vi "Prod - Uninitialize.vi"(8 "Error In":errorcluster, 11 "Prod-Data In":T2={"Queue_Producer"=refnum, "Queue_Consumer"=refnum, "To_GUI-Error_message"=refnum, "Rx-Data"=[], "Tx-Data"=[], "Console log"="", "Communication Settings"={"Tx Protocol"=enum."Not Active", "Rx Protocol"=enum."Serial", "Serial"={"Tx Port"="", "Rx Port"="", "Baud rate"=8, "Parity"=enum."Space", "Data bits"=0, "Stop bits"=0, "Flow control"=enum."None", "Tx Resource"="", "Rx Resource"=""}, "MIDI Device"={"Input uDevice ID"=0, "Output uDevice ID"=0, "hmidiout Handle"=0, "hmidiin Handle"=0}, "Bluetooth"={"Dummy"=""}, "USB"={"Dummy"=""}}, "MIDI-Messages"=[], "Queue_Session"=refnum, "To_GUI-Pre-Session"=refnum, "To_GUI-Producer"=refnum, "Tx Info"={"Datatype"=[], "Bytesize"=[], "Strings"=[], "ByteSum"=0}, "Payload"=variant, "Timout-Time[ms]"=0, "To_GUI-Session"=refnum, "CPU(ms)"=0}) -> (0 "Error Out":errorcluster, 3 "Prod-Data Out":T2={"Queue_Producer"=refnum, "Queue_Consumer"=refnum, "To_GUI-Error_message"=refnum, "Rx-Data"=[], "Tx-Data"=[], "Console log"="", "Communication Settings"={"Tx Protocol"=enum."Not Active", "Rx Protocol"=enum."Serial", "Serial"={"Tx Port"="", "Rx Port"="", "Baud rate"=8, "Parity"=enum."Space", "Data bits"=0, "Stop bits"=0, "Flow control"=enum."None", "Tx Resource"="", "Rx Resource"=""}, "MIDI Device"={"Input uDevice ID"=0, "Output uDevice ID"=0, "hmidiout Handle"=0, "hmidiin Handle"=0}, "Bluetooth"={"Dummy"=""}, "USB"={"Dummy"=""}}, "MIDI-Messages"=[], "Queue_Session"=refnum, "To_GUI-Pre-Session"=refnum, "To_GUI-Producer"=refnum, "Tx Info"={"Datatype"=[], "Bytesize"=[], "Strings"=[], "ByteSum"=0}, "Payload"=variant, "Timout-Time[ms]"=0, "To_GUI-Session"=refnum, "CPU(ms)"=0})   [LabVIEW 2019]
doc: "Initiates the producer based on IO settings."
uses:
  Controls/Producer-Data.ctl
  Common/Controls/Application_Message.ctl
  Common/Controls/Application_State.ctl
  Common/Controls/Communication_Settings.ctl
  Common/Controls/Communication_Protocols.ctl
  MIDI/Controls/MIDI-Message_Array.ctl
  MIDI/Controls/MIDI-Message_Cluster.ctl
  MIDI/Controls/Meta_Commands.ctl
  Controls/Prod - Tx_Info.ctl
  <vilib>/Utility/error.llb/DialogType.ctl
  winmm.dll
panel:
  in  "Control Tab":T1(tab)
  out "Console":string
  out "Error Message":string
  out "VI-filename":string
  out "VI Path":path
  out "Code Size":u32
  out "Revision Number":u32
  in  "Tool Bar:Visible":bool
  in  "Execution:Show Front Panel On Call":bool
  out "VI-Name":string
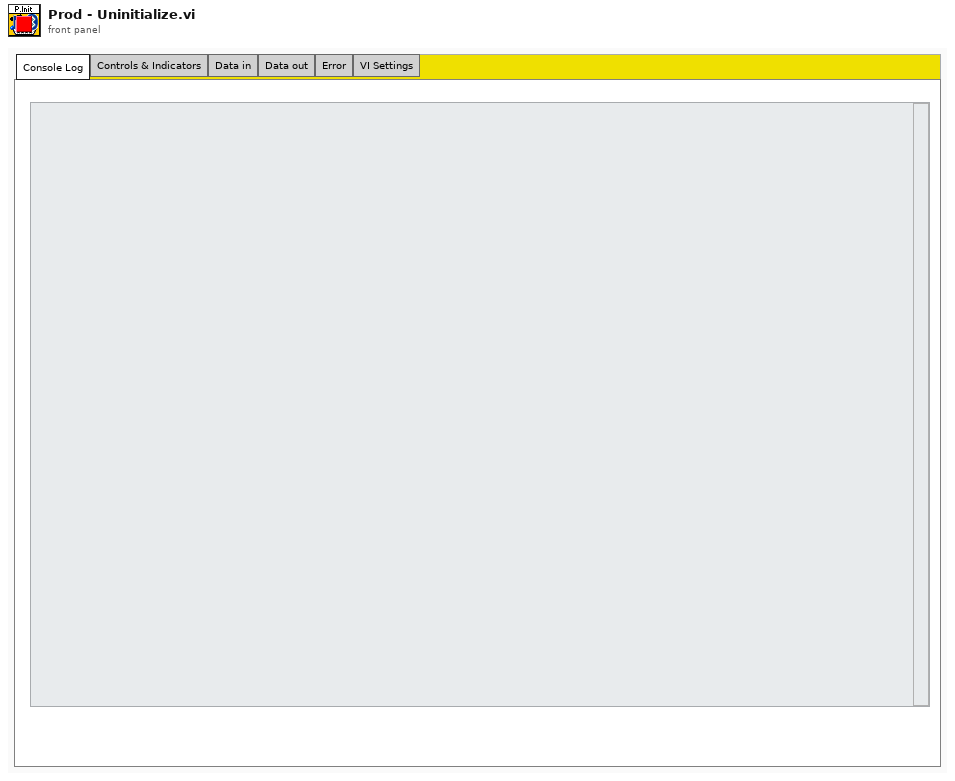
[diagram p1: front panel]
types:
  T1 = enum32{"Console Log", "Controls & Indicators", "Data in", "Data out", "Error", "VI Settings"}
  T2 = typedef "Producer-Data.ctl" = cluster{"Queue_Producer":refnum<queue>, "Queue_Consumer":refnum<queue>, "To_GUI-Error_message":refnum<user-event>, "Rx-Data":i8[], "Tx-Data":i8[], "Console log":string, "Communication Settings":T3, "MIDI-Messages":T5, "Queue_Session":refnum<queue>, "To_GUI-Pre-Session":refnum<user-event>, "To_GUI-Producer":refnum<user-event>, "Tx Info":T8, "Payload":variant, "Timout-Time[ms]":i32, "To_GUI-Session":refnum<user-event>, "CPU(ms)":u32}
  T3 = typedef "Communication_Settings.ctl" = cluster{"Tx Protocol":T4, "Rx Protocol":T4, "Serial":cluster{"Tx Port":refnum<visa-resource-name>, "Rx Port":refnum<visa-resource-name>, "Baud rate":i32, "Parity":enum16{"None", "Odd", "Even", "Mark", "Space"}, "Data bits":i32, "Stop bits":i32, "Flow control":enum16{"None", "XON/XOFF", "RTS/CTS", "XON/XOFF & RTS/CTS", "DTR/DSR", "XON/XOFF & DTR/DSR"}, "Tx Resource":refnum<visa-resource-name>, "Rx Resource":refnum<visa-resource-name>}, "MIDI Device":cluster{"Input uDevice ID":u32, "Output uDevice ID":u32, "hmidiout Handle":i32, "hmidiin Handle":i32}, "Bluetooth":cluster{"Dummy":string}, "USB":cluster{"Dummy":string}}
  T4 = typedef "Communication_Protocols.ctl" = enum16{"Serial", "Bluetooth", "USB-MIDI", "MIDI (Audio Device)", "Not Active"}
  T5 = typedef "MIDI-Message_Array.ctl" = T6[]
  T6 = typedef "MIDI-Message_Cluster.ctl" = cluster{"Message Name":string, "Meta value":i32, "Datastring":string, "Datatype":T7}
  T7 = typedef "Meta_Commands.ctl" = enum16{"No Data", "Pause", "Loop", "Wait for Rx", "Delay", "Break", "MIDI"}
  T8 = typedef "Prod - Tx_Info.ctl" = cluster{"Datatype":T7[], "Bytesize":i32[], "Strings":string[], "ByteSum":i32}
  T9 = typedef "DialogType.ctl" = u16
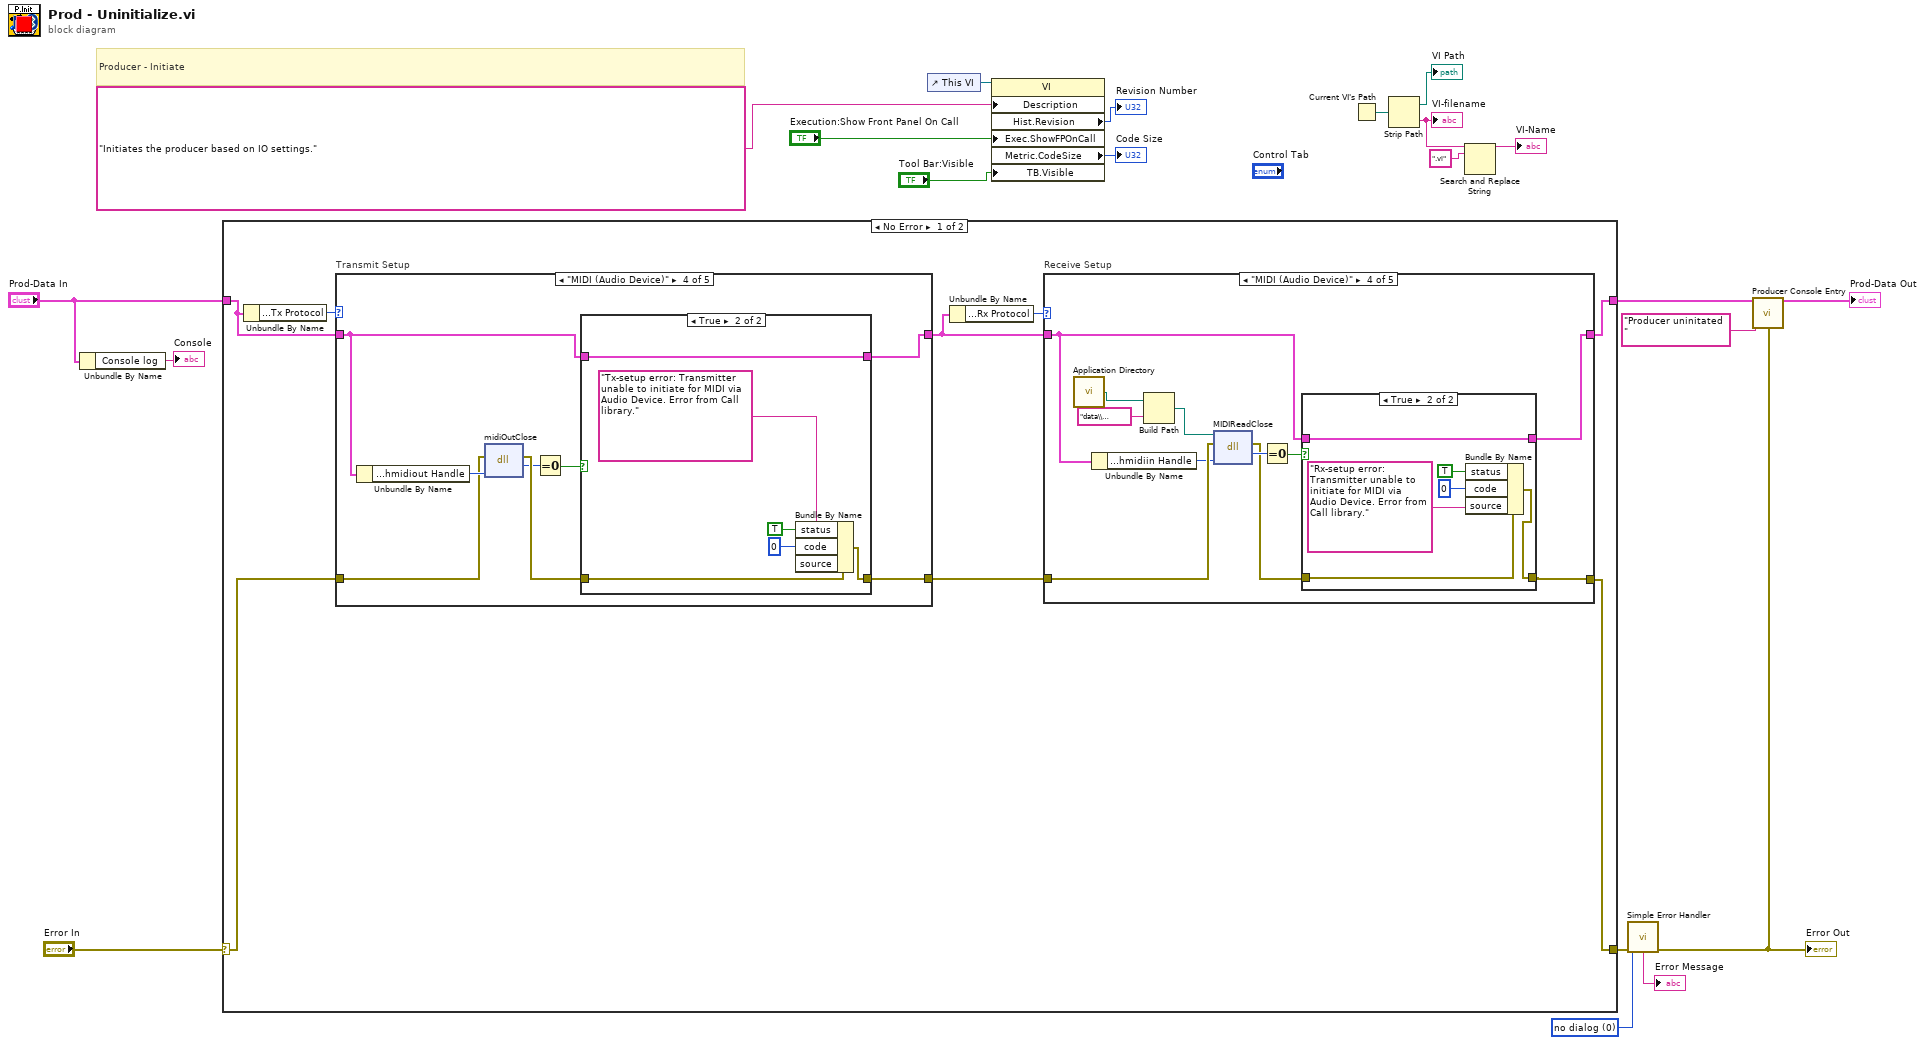
[diagram p0: block diagram]
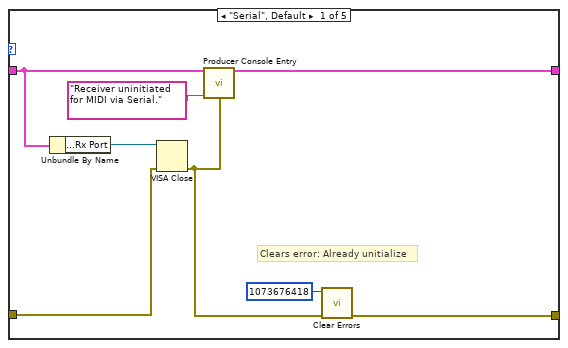
[diagram p2: hidden frame]
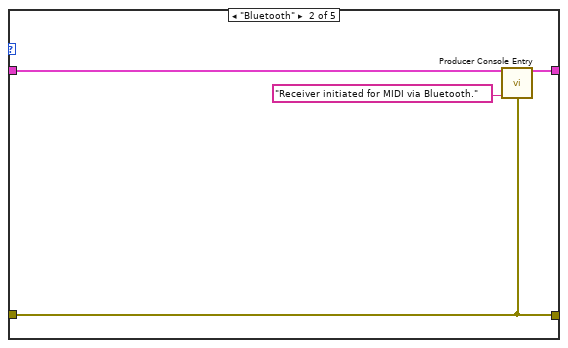
[diagram p3: hidden frame]
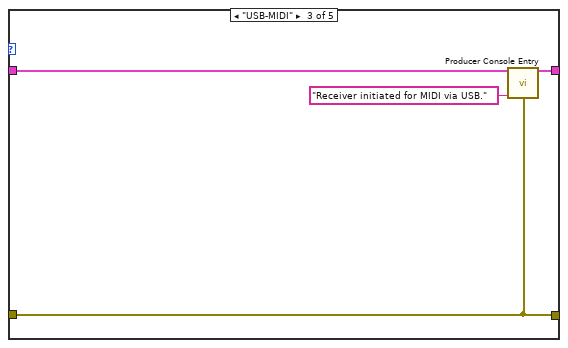
[diagram p4: hidden frame]
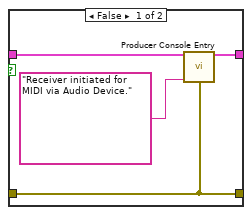
[diagram p5: hidden frame]
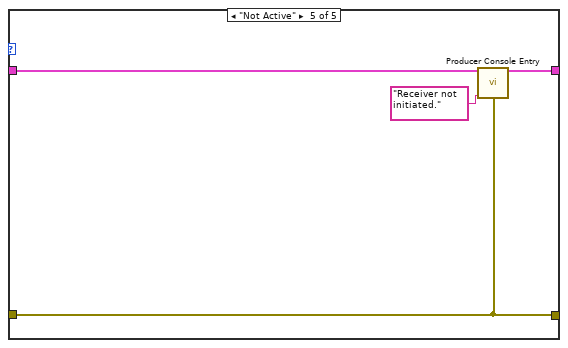
[diagram p6: hidden frame]
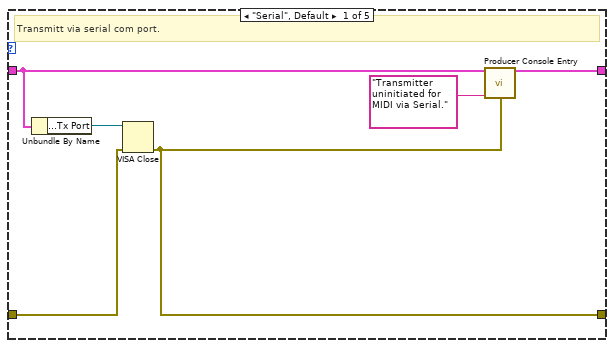
[diagram p7: hidden frame]
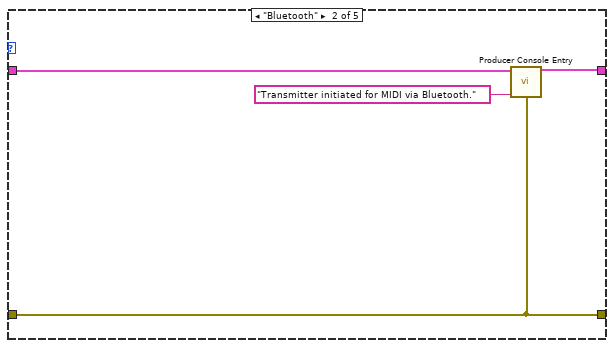
[diagram p8: hidden frame]
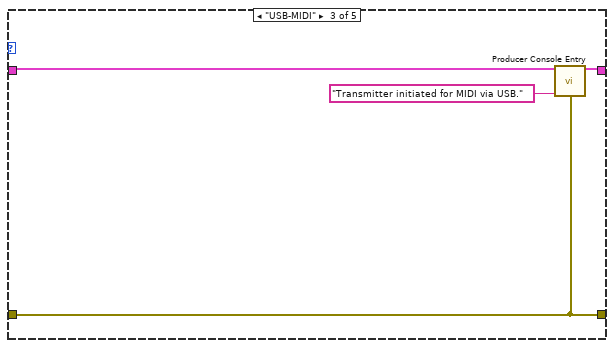
[diagram p9: hidden frame]
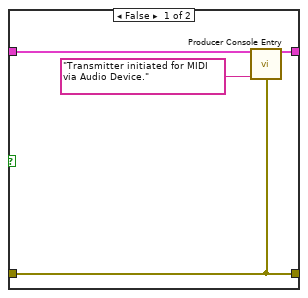
[diagram p10: hidden frame]
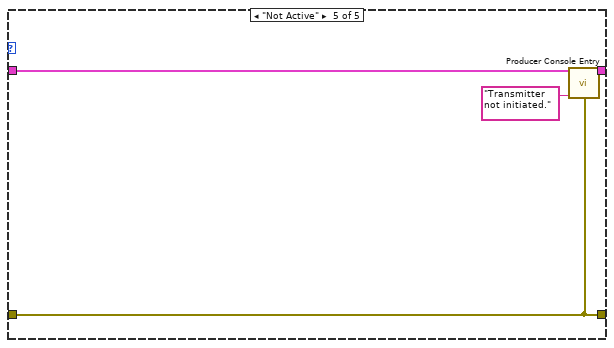
[diagram p11: hidden frame]
diagram:
  w4 = T9 0 items=["no dialog", "OK message", "continue or stop message", "OK message + warnings", "continue/stop + warnings"] ("type of dialog (OK msg:1)")
  # "Producer - Initiate"
  n1 = Unbundle By Name("Prod-Data In") -> ("Console log"=→"Console":string)
  n2 = case shown="No Error" "Error In" {
    selector: "Error In" -> [w24 w108]
    tunnel: [w22 w108] -> w6
    tunnel: "Prod-Data In" -> [w28 w107]
    tunnel: [w25 w107] -> w7
    frame No Error {
      n3 = Unbundle By Name(w28) -> ("Communication Settings.Tx Protocol"=w29:T4)
      n4 = case "Transmit Setup" shown="\"MIDI (Audio Device)\"" w29 {
        tunnel: w28 -> [w76 w78 w82 w85 w105]
        tunnel: [w75 w80 w83 w86 w106] -> w26
        tunnel: w24 -> [w72 w79 w81 w91 w103]
        tunnel: [w71 w79 w81 w89 w103] -> w23
        frame "Serial", Default {
          # "Transmitt via serial com port."
          n5 = Unbundle By Name(w76) -> ("Communication Settings.Serial.Tx Port"=w73:refnum<visa-resource-name>)
          n6 = VISA Close(VISA resource name=w73, error in (no error)=w72) -> (error out=w71:errorcluster)
          n7 = call "Producer Console Entry.vi"("Prod-Data In"=w76, "Console Entry"="Transmitter uninitiated for MIDI via Serial.", "Error In"=w71) -> ("Prod-Data Out"=w75:T2)  [unwired: 12 in]
        }
        frame "Bluetooth" {
          n8 = call "Producer Console Entry.vi"("Prod-Data In"=w78, "Console Entry"="Transmitter initiated for MIDI via Bluetooth.", "Error In"=w79) -> ("Prod-Data Out"=w80:T2)  [unwired: 12 in]
        }
        frame "USB-MIDI" {
          n9 = call "Producer Console Entry.vi"("Prod-Data In"=w82, "Console Entry"="Transmitter initiated for MIDI via USB.", "Error In"=w81) -> ("Prod-Data Out"=w83:T2)  [unwired: 12 in]
        }
        frame "MIDI (Audio Device)" {
          n10 = Unbundle By Name(w85) -> ("Communication Settings.MIDI Device.hmidiout Handle"=w92:i32)
          n11 = dll-call lib="winmm.dll" fn="midiOutClose"(error in=w91, "hmidiout"=w92) -> (error out=w90:errorcluster, w88:i32)  [unwired: 3 in, 1 out]
          n12 = Equal To 0?(x=w88) -> (x = 0?=w87:bool)
          n13 = case shown="True" w87 {
            tunnel: w90 -> [w96 w102]
            tunnel: [w96 w98] -> w89
            tunnel: [w94 w97] -> w86
            tunnel: w85 -> [w93 w97]
            frame False {
              n14 = call "Producer Console Entry.vi"("Prod-Data In"=w93, "Console Entry"="Transmitter initiated for MIDI via Audio Device.", "Error In"=w96) -> ("Prod-Data Out"=w94:T2)  [unwired: 12 in]
            }
            frame True {
              n15 = Bundle By Name(cluster=w102, "status"=TRUE, "code"=0, "source"="Tx-setup error: Transmitter unable to initiate for MIDI via Audio Device. Error from Call library.") -> (w98:errorcluster)
            }
          }
        }
        frame "Not Active" {
          n16 = call "Producer Console Entry.vi"("Prod-Data In"=w105, "Console Entry"="Transmitter not initiated.", "Error In"=w103) -> ("Prod-Data Out"=w106:T2)  [unwired: 12 in]
        }
      }
      n17 = Unbundle By Name(w26) -> ("Communication Settings.Rx Protocol"=w27:T4)
      n18 = case "Receive Setup" shown="\"MIDI (Audio Device)\"" w27 {
        tunnel: w26 -> [w36 w39 w43 w50 w69]
        tunnel: [w34 w40 w44 w49 w70] -> w25
        tunnel: w23 -> [w33 w38 w42 w56 w68]
        tunnel: [w31 w38 w42 w51 w68] -> w22
        frame "Serial", Default {
          # "Clears error: Already unitialize"
          n19 = Unbundle By Name(w36) -> ("Communication Settings.Serial.Rx Port"=w37:refnum<visa-resource-name>)
          n20 = VISA Close(VISA resource name=w37, error in (no error)=w33) -> (error out=w32:errorcluster)
          n21 = call "Producer Console Entry.vi"("Prod-Data In"=w36, "Console Entry"="Receiver uninitiated for MIDI via Serial.", "Error In"=w32) -> ("Prod-Data Out"=w34:T2)  [unwired: 12 in]
          n22 = call <vilib>:"Clear Errors.vi"("error in (no error)"=w32, "specific error code to clear (0: all)"=1073676418) -> ("error out"=w31:errorcluster)  [unwired: 4 in, 1 out]
        }
        frame "Bluetooth" {
          n23 = call "Producer Console Entry.vi"("Prod-Data In"=w39, "Console Entry"="Receiver initiated for MIDI via Bluetooth.", "Error In"=w38) -> ("Prod-Data Out"=w40:T2)  [unwired: 12 in]
        }
        frame "USB-MIDI" {
          n24 = call "Producer Console Entry.vi"("Prod-Data In"=w43, "Console Entry"="Receiver initiated for MIDI via USB.", "Error In"=w42) -> ("Prod-Data Out"=w44:T2)  [unwired: 12 in]
        }
        frame "MIDI (Audio Device)" {
          n25 = call <vilib>:"Application Directory.vi"() -> ("Application Directory"=w48:path)
          n26 = Unbundle By Name(w50) -> ("Communication Settings.MIDI Device.hmidiin Handle"=w55:i32)
          n27 = Build Path(base path=w48, name or relative path="data\\MIDIDLL.dll") -> (appended path=w46:path)
          n28 = dll-call lib="C:/Users/bjerk/OneDrive/Jobb/Nordic Semiconductor/MIDI Development Tool/data/MIDIDLL.dll" fn="MIDIReadClose"(path in=w46, error in=w56, "hmidiin"=w55) -> (error out=w52:errorcluster, "return type"=w54:i32)  [unwired: 2 in, 1 out]
          n29 = Equal To 0?(x=w54) -> (x = 0?=w53:bool)
          n30 = case shown="True" w53 {
            tunnel: w52 -> [w60 w62]
            tunnel: [w60 w61] -> w51
            tunnel: w50 -> [w59 w63]
            tunnel: [w57 w63] -> w49
            frame False {
              n31 = call "Producer Console Entry.vi"("Prod-Data In"=w59, "Console Entry"="Receiver initiated for MIDI via Audio Device.", "Error In"=w60) -> ("Prod-Data Out"=w57:T2)  [unwired: 12 in]
            }
            frame True {
              n32 = Bundle By Name(cluster=w62, "status"=TRUE, "code"=0, "source"="Rx-setup error: Transmitter unable to initiate for MIDI via Audio Device. Error from Call library.") -> (w61:errorcluster)
            }
          }
        }
        frame "Not Active" {
          n33 = call "Producer Console Entry.vi"("Prod-Data In"=w69, "Console Entry"="Receiver not initiated.", "Error In"=w68) -> ("Prod-Data Out"=w70:T2)  [unwired: 12 in]
        }
      }
    }
    frame Error {
    }
  }
  n34 = control-ref of="This VI"() -> (w14:refnum<vi>)
  n35 = property class="VI"(reference=w14, "Description"="Initiates the producer based on IO settings.", "Exec.ShowFPOnCall"="Execution:Show Front Panel On Call", "TB.Visible"="Tool Bar:Visible") -> ("Hist.Revision"=→"Revision Number":u32, "Metric.CodeSize"=→"Code Size":u32)  [unwired: 1 in, 2 out]
  n36 = Current VI's Path() -> (path=w21:path)
  n37 = Strip Path(path=w21) -> (stripped path=→"VI Path":path, name=w11:string)
  "VI-filename" <- w11
  n38 = Search and Replace String(input string=w11, search string=".vi") -> (result string=→"VI-Name":string)  [unwired: 6 in, 3 out]
  n39 = call <vilib>:"Simple Error Handler.vi"("type of dialog (OK msg:1)"=w4, "error in (no error)"=w6) -> ("error out"=w5:errorcluster, "message"=→"Error Message":string)  [unwired: 3 in, 3 out]
  "Error Out" <- w5
  n40 = call "Producer Console Entry.vi"("Prod-Data In"=w7, "Console Entry"="Producer uninitated ", "Error In"=w5) -> ("Prod-Data Out"=→"Prod-Data Out":T2)  [unwired: 12 in]
